vi "Value Entry_STR.vi"(11 "Value In":string) -> (2 "Apply":bool, 3 "Value Out":string)   [LabVIEW 2018, in "Tag Watchlist.lvlib"]
uses:
  Tag Watchlist.lvlib
panel:
  in  "Value":string caption="New Value"
  in  "Cancel":bool
  in  "OK":bool
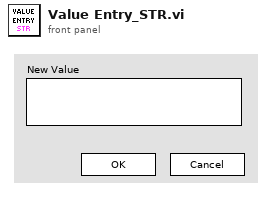
[diagram p1: front panel]
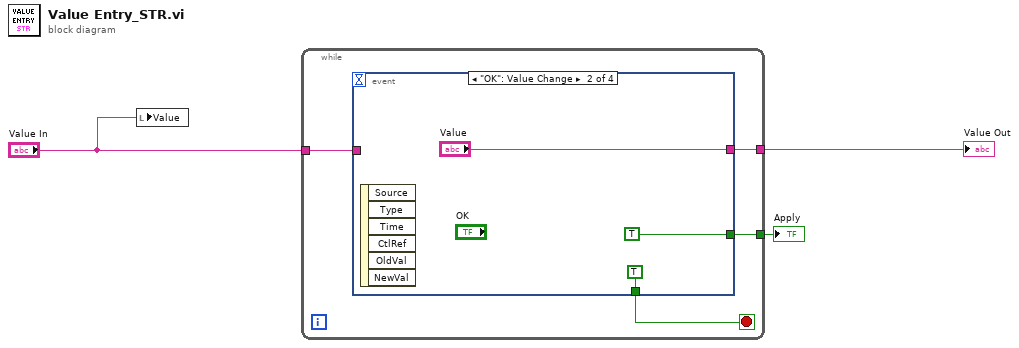
[diagram p0: block diagram]
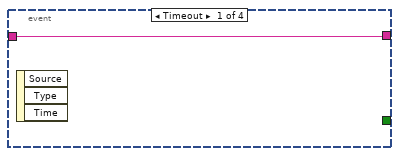
[diagram p2: hidden frame]
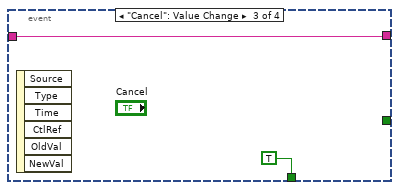
[diagram p3: hidden frame]
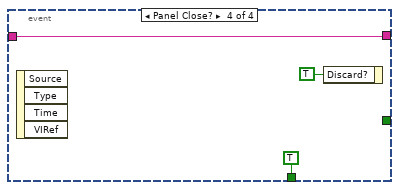
[diagram p4: hidden frame]
diagram:
  n1 = local write "Value"("Value In") -> ()
  n2 = while {
    tunnel: "Value In" -> [w7]
    tunnel: [w6] -> w2
    tunnel: [w4] -> w1
    stop <- w5 stop-if-true
    n3 = event shown="[1] \"OK\": Value Change" {
      selector: _ -> [_ _ _ _]
      dyn-events: _ -> [_ _ _ _]
      timeout: _ -> [_ _ _ _]
      tunnel: w7 -> [w8 _ w12 w14]
      tunnel: [w8 "Value" w12 w14] -> w6
      tunnel: [_ TRUE TRUE TRUE] -> w5
      tunnel: [_ TRUE _ _] -> w4
      event Timeout {
        n4 = event-data() -> ()  [unwired: 1 in, 3 out]
      }
      event "OK": Value Change {
        n5 = event-data() -> ()  [unwired: 1 in, 6 out]
      }
      event "Cancel": Value Change {
        n6 = event-data() -> ()  [unwired: 1 in, 6 out]
      }
      event Panel Close? {
        n7 = event-data() -> ()  [unwired: 1 in, 4 out]
        n8 = event-data("Discard?"=TRUE) -> ()  [unwired: 1 in, 1 out]
      }
    }
  }
  "Value Out" <- w2
  "Apply" <- w1
